vi "Main Page.vi"(8 "error in (no error)":errorcluster, 11 "Node Ptr":T1 format="%.0x") -> (0 "error out":errorcluster)   [LabVIEW 2019, in "SLSC EDS System Explorer.lvlib"]
uses:
  SLSC EDS System Explorer.lvlib
  <vilib>/NI VeriStand/Custom Device API/Custom Device Item Ref.ctl
  <vilib>/Utility/error.llb/DialogType.ctl
  <vilib>/Utility/miscctls.llb/LVStringsAndValuesArrayTypeDef_U16.ctl
  Shared/Constants.vi
  <vilib>/NI VeriStand/Custom Device API/Set Item Property (Variant).vi
  <vilib>/SLSC/Initialize Session with Devices.vi
  <vilib>/SLSC/Close Session.vi
  <vilib>/NI VeriStand/Custom Device API/Custom Device API.lvlib
  Shared/SLSC EDS Shared.lvlib
  SLSC UI API/SLSC Tree Control.lvlib
  SLSC CD API/SLSC CD System Explorer/SLSC CD System Explorer.lvlib
  Engine/SLSC EDS Engine.lvlib
  <vilib>/SLSC/SLSC.lvlib
  SLSC EDS API/SLSC EDS API.lvlib
  SLSC CD API/SLSC CD Engine/SLSC CD Engine.lvlib
panel:
  out "Custom Device State":string
  in  "Refresh page":bool
  out "SLSC Device Name":string
  out "State":u16(ring) items=["Not Configured", "Basic Configured"]
  out "Module Name":string
  in  "Help Button":bool
  out "Slot Number":i32
  out "CD Version":string caption="Version"
  in  "Header":cluster{"Section Name":string}={"Section Name"="SLSC EDS Custom Device"}
  in  "Name":string
  in  "SHDocVw.IWebBrowser":refnum<k7>(container)
  in  "Description":string
  in  "Modify Reset Value?":bool
  in  "I8":i8
  in  "U8":u8 format="%.0x"
  in  "I32":i32
  in  "U32":u32 format="%.0x"
  in  "U64":u64 format="%.0x"
  in  "I64":i64
  in  "DBL":dbl format="%#_16g"
  in  "Ring":u16(ring)
  in  "Add":bool
  in  "Remove":bool
  in  "Header 2":cluster{"Section Name":string}={"Section Name"="Custom Device Item Settings"}
  in  "Property tree":string[](tree)
  in  "Loop rate":u32
  in  "Apply Reset":bool
  in  "Apply Default":bool
  # "ms"
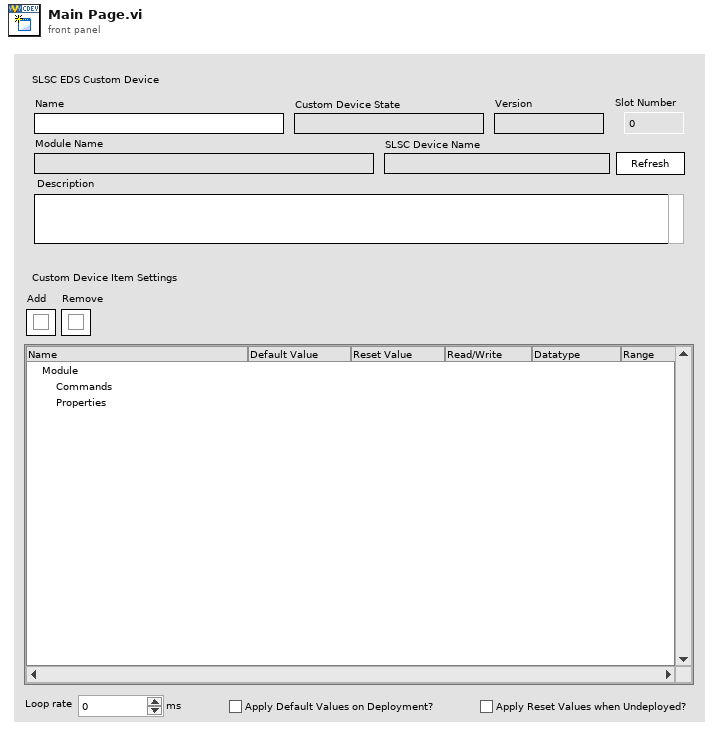
[diagram p1: front panel]
types:
  T1 = typedef "Custom Device API.lvlib/Custom Device Item Ref.ctl" = u64
  T2 = typedef "EDSjsonStructure.ctl" = cluster{"vendorNum":u32, "vendorName":string, "vendorPrefix":string, "productNum":u32, "productName":string, "capsVersion":string, "capsSpecVersion":u32, "capsSpecOldestCompatibleVersion":u32, "enums":T3[], "properties":T4[], "commands":T5[], "scales":T6[], "physicalChannels":T7[], "registerMap":cluster{"registers":T8[]}}
  T3 = typedef "enum.ctl" = cluster{"name":string, "description-en":string, "values":cluster{"name":string, "description-en":string, "value":i32}[]}
  T4 = typedef "property.ctl" = cluster{"name":string, "description-en":string, "documentation-en":string, "dataType":string, "bitfield":string, "access":string, "scale":string, "value":variant, "min":variant, "max":variant, "default value":variant}
  T5 = typedef "command.ctl" = cluster{"name":string, "description-en":string, "documentation-en":string, "startBitfield":string, "waitTimeInMs":i32, "doneBitfield":string, "doneInterrupt":string, "doneTimeoutInMs":i32, "value":variant}
  T6 = typedef "scale.ctl" = cluster{"name":string, "description-en":string, "m":dbl, "b":dbl, "forwardCoeffs":dbl[], "reverseCoeffs":dbl[], "coercion":string, "table":cluster{"scaled":dbl, "unscaled":dbl}[]}
  T7 = typedef "physicalChannel.ctl" = cluster{"name":string, "description-en":string, "commands":T5[], "properties":T4[]}
  T8 = typedef "register.ctl" = cluster{"name":string, "description-en":string, "access":string, "address":u32, "size":u32, "bitfields":cluster{"name":string, "description-en":string, "offset":u32, "size":u32, "signed":bool, "strobe":bool}[]}
  T9 = cluster{"Left Cell String":string, "Child Text":string[], "Child Tag":string, "Item Indent":i32, "Child Only?":bool, "Glyph Index":i32}[]
  T10 = typedef "LVStringsAndValuesArrayTypeDef_U16.ctl" = cluster{"String":string, "Value":u16}[]
  T11 = typedef "Custom Device API.lvlib/Custom Device Commands.ctl" = enum16{"Default", "Item renamed", "Shutdown", "Dynamic button pressed"}
  T12 = typedef "Custom Device API.lvlib/Custom Device Item Info.ctl" = cluster{"Name":string, "Is Channel":bool, "GUID":string, "Is Waveform":bool}
  T13 = typedef "DialogType.ctl" = u16
  T14 = typedef "SLSC EDS Shared.lvlib/SLSC Static Settings.ctl" = cluster{"Properties":cluster{"Boolean Properties":cluster{"property":refnum<k21>, "Value":bool, "SLSC Item":refnum<k21>, "reset value":bool}[], "Double Properties":cluster{"property":refnum<k21>, "Double Write":dbl, "SLSC Item":refnum<k21>, "Double Reset Value":dbl}[], "I32 Properties":cluster{"property":refnum<k21>, "Int32 Write":i32, "SLSC Item":refnum<k21>, "Int32 Reset Value":i32}[], "I64 Properties":cluster{"property":refnum<k21>, "Int64 Write":i64, "SLSC Item":refnum<k21>, "Int64 Reset Value":i64}[], "String Properties":cluster{"property":refnum<k21>, "String Write":string, "SLSC Item":refnum<k21>, "String Reset Value":string}[], "U32 Properties":cluster{"property":refnum<k21>, "UInt32 Write":u32, "SLSC Item":refnum<k21>, "UInt32 Reset Value":u32}[], "U64 Properties":cluster{"property":refnum<k21>, "UInt64 Write":u64, "SLSC Item":refnum<k21>, "UInt64 Reset Value":u64}[]}, "Commands":T15[], "Reset Commands":T15[], "Apply Values on Deployment":bool, "Apply Reset on Undeployment":bool, "Change Commands":T15[]}
  T15 = typedef "SLSC CD Shared.lvlib/SLSC Dynamic Channel.ctl" = cluster{"SLSC Item":string, "property":string, "Data Type":T16}
  T16 = typedef "SLSC CD Shared.lvlib/SLSC Datatype.ctl" = enum16{"Bool", "Double", "I32", "I64", "String", "U32", "U64"}
  T17 = typedef "SLSC CD Shared.lvlib/SLSC Identification.ctl" = cluster{"vendorName":string, "productNum":u32, "capsVersion":string, "capsSpecVersion":u32, "productName":string, "vendorNum":u32, "vendorPrefix":string, "capsSpecOldestCompatibleVersion":u32}
  T18 = cluster{"Left Cell String":string, "Child Text":string[], "Child Tag":string, "Item Indent":i32, "Child Only?":bool, "Glyph Index":i32}
  T19 = cluster{"name":string, "description-en":string, "value":i32}[]
  T20 = typedef "LVPoint32TypeDef.ctl" = cluster{"Horizontal":i32, "Vertical":i32}
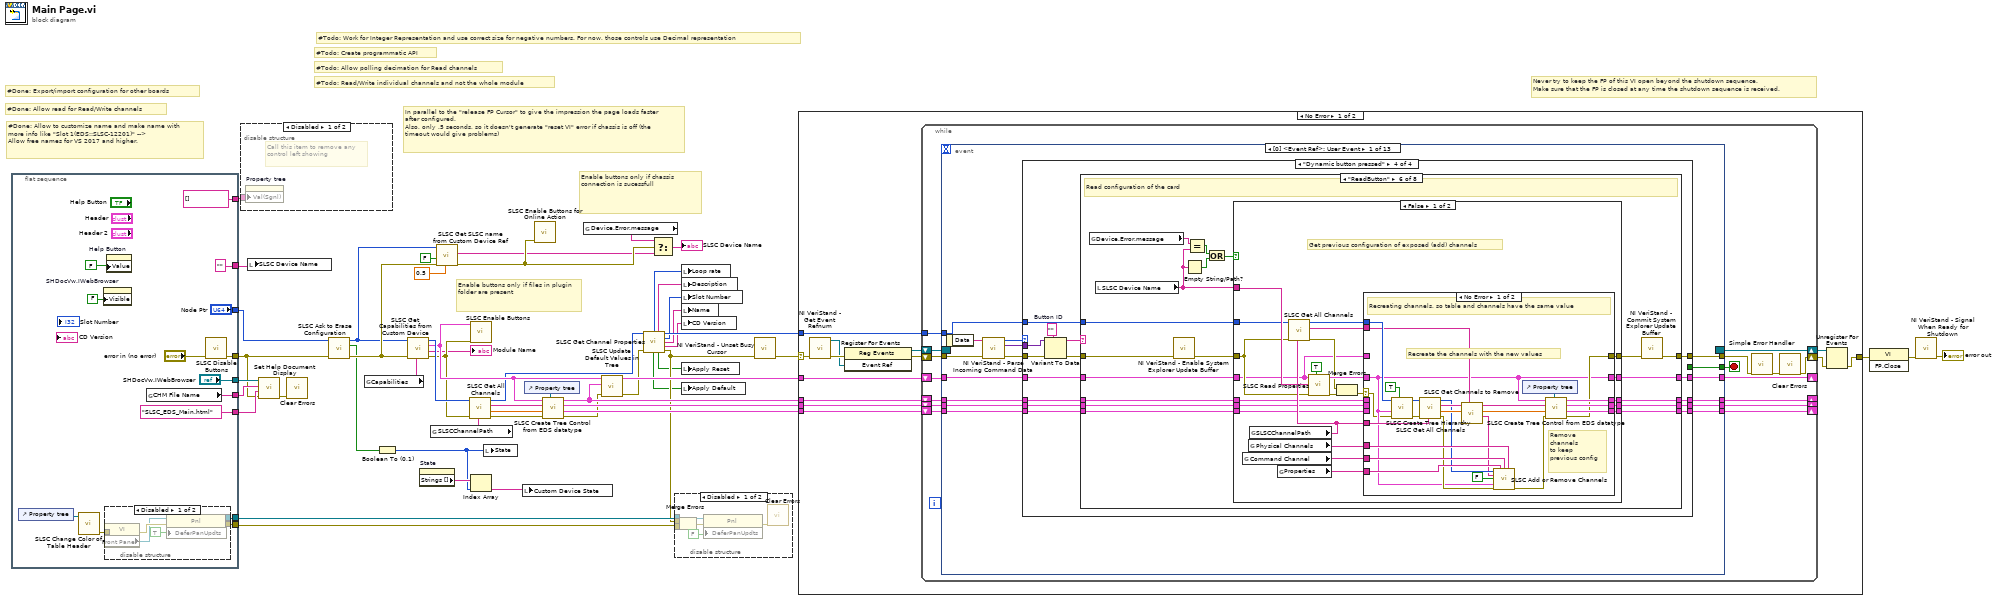
[diagram p0: block diagram]
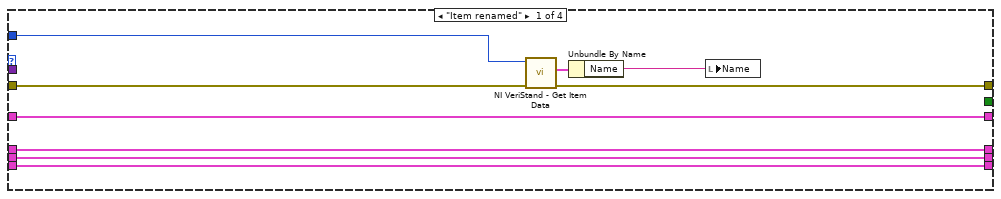
[diagram p5: hidden frame]
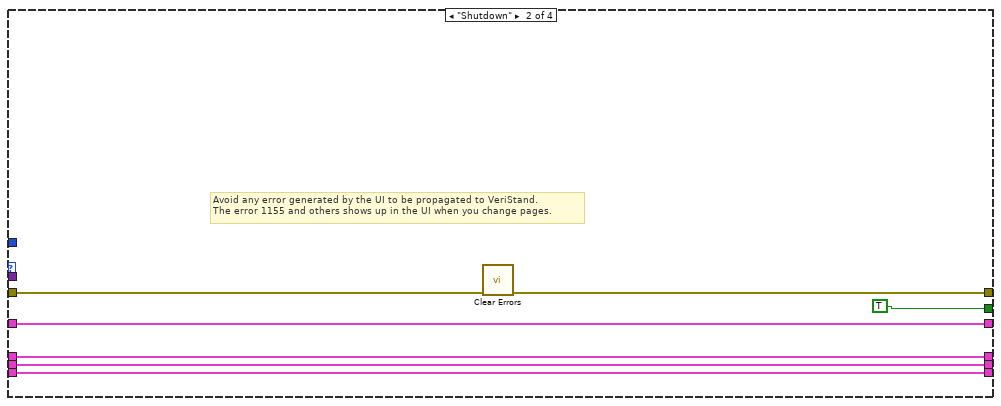
[diagram p6: hidden frame]
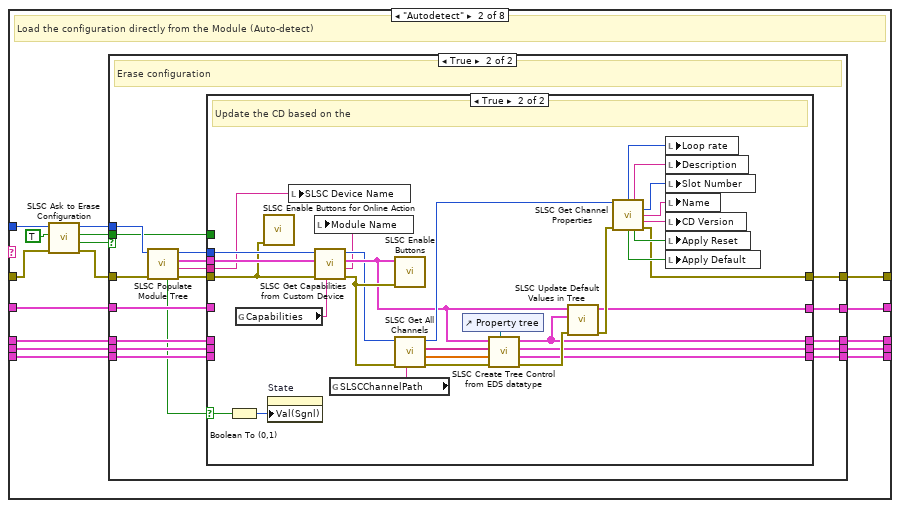
[diagram p9: hidden frame]
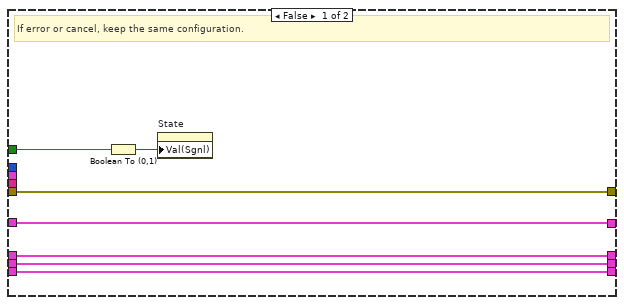
[diagram p11: hidden frame]
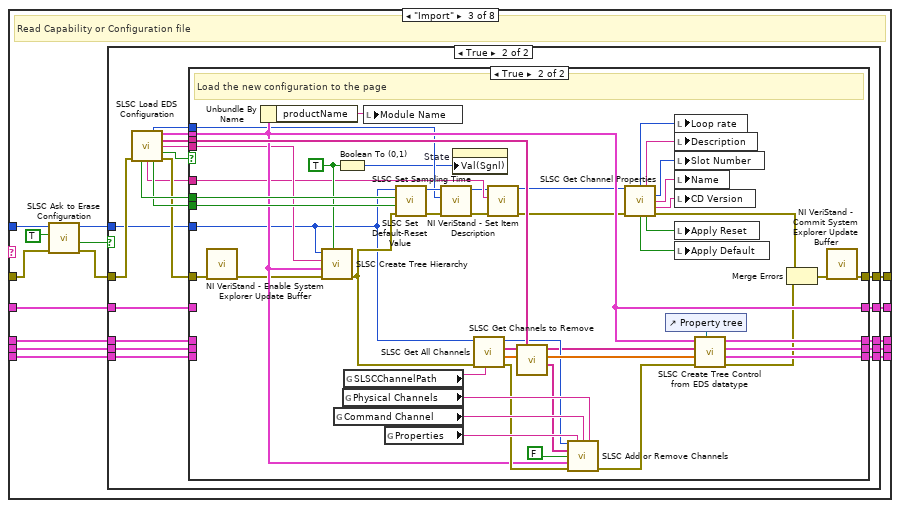
[diagram p12: hidden frame]
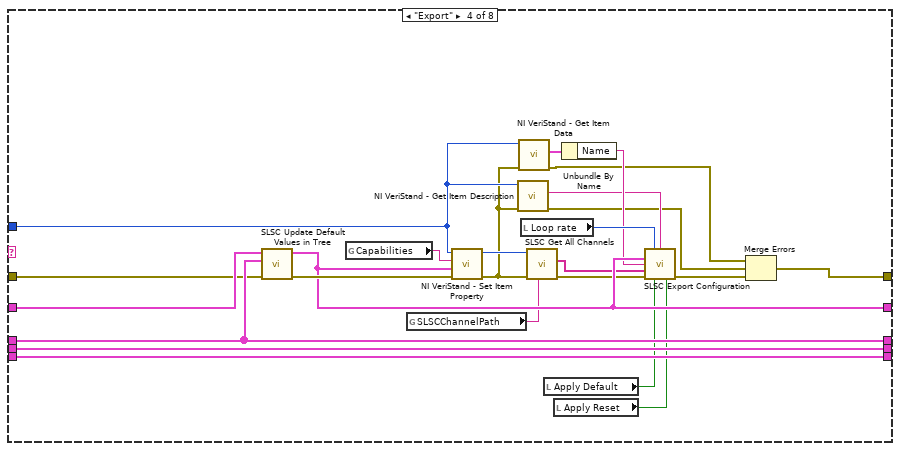
[diagram p15: hidden frame]
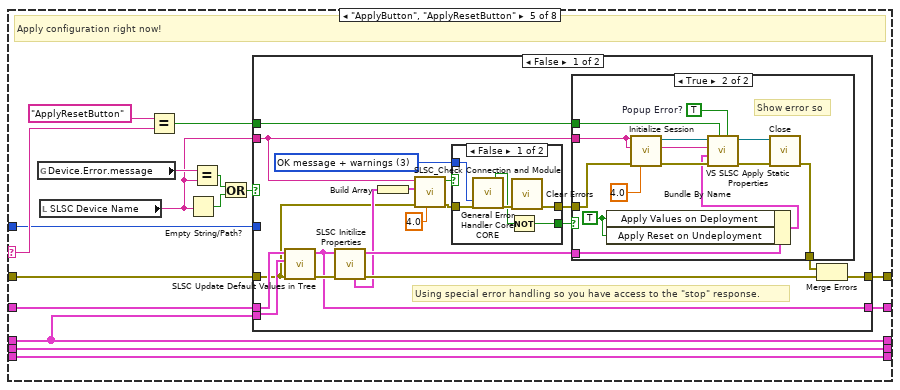
[diagram p16: hidden frame]
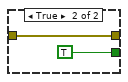
[diagram p18: hidden frame]
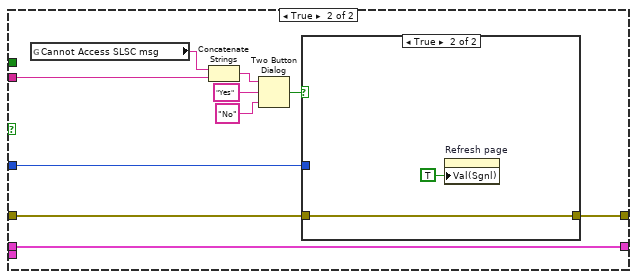
[diagram p19: hidden frame]
diagram:
  # "Enable buttons only if files in plugin folder are present"
  # "Enable buttons only if chassis connection is sucessfull"
  # "#Todo: Work for Integer Representation and use correct size for negative numbers. For now, those controls use Decimal representation"
  # "#Done: Allow to customize name and make name with more info like \"Slot 1(EDS::SLSC-12201)\" --> \nAllow free names for VS 2017 and higher."
  # "#Todo: Read/Write individual channels and not the whole module"
  # "In parallel to the \"release FP Cursor\" to give the impression the page loads faster after configured. \nAlso, only .5 seconds, so it doesn't generate \"reset VI\" error if chassis is off (the timeout would give problems)"
  # "Never try to keep the FP of this VI open beyond the shutdown sequence.\nMake sure that the FP is closed at any time the shutdown sequence is received."
  # "#Todo: Allow polling decimation for Read channels"
  # "#Done: Allow read for Read/Write channels"
  # "#Todo: Create programmatic API"
  # "#Done: Export/import configuration for other boards"
  n1 = flat-sequence {
    tunnel: ["Node Ptr"] -> w10
    tunnel: [w53] -> w11
    tunnel: ["SHDocVw.IWebBrowser"] -> w50
    tunnel: ["SLSC_EDS_Main.html" ("HTML File")] -> w49
    tunnel: [w63] -> w48
    tunnel: [string[] [] ("Property tree")] -> w43
    tunnel: ["" ("SLSC Module Name")] -> w42
    tunnel: [w57] -> w31
    tunnel: [w56] -> w30
    frame #0 {
      n2 = control-ref of="Property tree"() -> (w55:refnum<vi>)
      n3 = call "SLSC Change Color of Table Header.vi"("TreeControl in"=w55) -> ("error out"=w54:errorcluster)  [unwired: 10 in]
      n4 = property on="SHDocVw.IWebBrowser" class="AXCont"("Visible"=FALSE) -> ()  [unwired: 2 in, 2 out]
      n5 = disable-structure shown="Disabled" {
        disable-tunnel: [w70 _] -> w57
        disable-tunnel: [w69 _] -> w56
        disable-tunnel: w54 -> [w67 _]
        frame Disabled {
          n6 = property class="VI"(error in=w67) -> (error out=w72:errorcluster, "Front Panel"=w68:refnum<vi>)  [unwired: 1 in, 1 out]
          n7 = property class="Pnl"(reference=w68, error in=w72, "DeferPanUpdts"=TRUE ("Defer Panel Updates")) -> (reference out=w70:refnum<vi>, error out=w69:errorcluster)
        }
        frame Enabled {
        }
      }
      n8 = property on="Help Button" class="Bool (strict)"("Value"=FALSE ("Visible")) -> ()  [unwired: 2 in, 2 out]
      n9 = global read "Constants.vi" "CHM File Name"() -> (w63:string)
      n10 = call "SLSC Disable Buttons.vi"("error in (no error)"="error in (no error)") -> ("error out"=w53:errorcluster)  [unwired: 10 in]
    }
  }
  n11 = disable-structure shown="Disabled" {
    disable-tunnel: w43 -> [w73 _]
    frame Disabled {
      # "Call this item to remove any control left showing"
      n12 = property on="Property tree" class="Tree (strict)"("Val(Sgnl)"=w73) -> ()  [unwired: 2 in, 2 out]
    }
    frame Enabled {
    }
  }
  n13 = local write "SLSC Device Name"(w42) -> ()
  n14 = call "Set Help Document Display.vi"("error in (no error)"=w11, "HTML File"=w49, "Main CHM File"=w48, "SHDocVw.IWebBrowser2"=w50) -> ("error out"=w29:errorcluster)  [unwired: 7 in]
  n15 = call <vilib>:"Clear Errors.vi"("error in (no error)"=w29) -> ()  [unwired: 1 in, 6 out]
  n16 = call "SLSC Ask to Erase Configuration.vi"("error in (no error)"=w11, "Device Item Ref in"=w10) -> ("error out"=w41:errorcluster, "initialized?"=w9:bool, "Item Ref out"=w40:T1)  [unwired: 6 in, 1 out]
  n17 = global read "Constants.vi" "Capabilities"() -> (w32:string)
  n18 = Boolean To (0,1)(Boolean=w9) -> (0, 1=w2:i16)
  n19 = call "SLSC Get Capabilities from Custom Device.vi"("Property Name"=w32, "error in (no error)"=w41, "Device Item Ref in"=w40) -> ("error out"=w28:errorcluster, "Product Name"=→"Module Name":string, "data"=w34:T2, "Item Ref out"=w38:T1)  [unwired: 3 in, 2 out]
  n20 = property on="State" class="Ring (strict)"() -> ("Strings []"=w3:string[])  [unwired: 2 in, 2 out]
  n21 = global read "Constants.vi" "SLSCChannelPath"() -> (w33:string)
  n22 = call "SLSC Get SLSC name from Custom Device Ref.vi"("connect timeout"=0.5, "error in (no error)"=w41, "Wait for mDSN?"=FALSE, "Item Ref in"=w40) -> ("error out"=w15:errorcluster, "SLSC Module Name"=w14:string)  [unwired: 4 in, 2 out]
  n23 = call "SLSC Get All Channels.vi"("SLSCChannelPath"=w33, "error in (no error)"=w28, "Item Ref in"=w38) -> ("error out"=w37:errorcluster, "Channel Values"=w35:dbl[], "TreeItem Channels"=w36:string[], "Item Ref out"=w16:T1)  [unwired: 5 in]
  n24 = call "SLSC Enable Buttons.vi"("error in (no error)"=w28, "data"=w34) -> ()  [unwired: 10 in]
  n25 = Index Array(array=w3, index=w2) -> (element=w1:string)
  n26 = local write "State"(w2) -> ()
  n27 = local write "Custom Device State"(w1) -> ()
  n28 = control-ref of="Property tree"() -> (w39:refnum<vi>)
  n29 = call "SLSC Enable Buttons for Online Action.vi"("error in (no error)"=w15) -> ()  [unwired: 11 in]
  n30 = call "SLSC Create Tree Control from EDS datatype.vi"("Property Tree"=w39, "error in (no error)"=w37, "Channel Values"=w35, "Properties to enable"=w36, "SLSC EDS module"=w34) -> ("error out"=w24:errorcluster, "Enum Strings"=w44:cluster{"name":string, string}[], "Enums"=w45:T3[], "SLSC Output Tree"=w46:T9)  [unwired: 3 in]
  n31 = global read "Constants.vi" "Device.Error.message"() -> (w12:string)
  n32 = call "SLSC Update Default Values in Tree.vi"("error in (no error)"=w24, "SLSC Output Tree"=w46, "SLSC EDS module in"=w34) -> ("error out"=w23:errorcluster, "SLSC EDS module out"=w47:T2)  [unwired: 7 in]
  n33 = call "SLSC Get Channel Properties.vi"("Node Ptr"=w16, "error in (no error)"=w23) -> ("Loop time (ms)"=w17:u32, "Description"=w19:string, "Section Ref out"=w22:T1, "Module Number"=w6:i32, "Name"=w18:string, "Device Version"=w5:string, "Default Value"=w21:bool, "Reset Value"=w20:bool, "error out"=w25:errorcluster)  [unwired: 5 in]
  n34 = Select(t=w12, s=w15, f=w14) -> (s? t:f=→"SLSC Device Name":string)
  n35 = disable-structure shown="Disabled" {
    disable-tunnel: w31 -> [w77 _]
    disable-tunnel: w30 -> [w76 _]
    disable-tunnel: w25 -> [w75 _]
    frame Disabled {
      n36 = Merge Errors(w75, w76) -> (w78:errorcluster)
      n37 = property class="Pnl"(reference=w77, error in=w78, "DeferPanUpdts"=FALSE ("Defer Panel Updates")) -> (error out=w74:errorcluster)  [unwired: 1 out]
      n38 = call <vilib>:"Clear Errors.vi"("error in (no error)"=w74) -> ()  [unwired: 1 in, 6 out]
    }
    frame Enabled {
    }
  }
  n39 = local write "Loop rate"(w17) -> ()
  n40 = local write "Description"(w19) -> ()
  n41 = local write "Slot Number"(w6) -> ()
  n42 = local write "Name"(w18) -> ()
  n43 = local write "CD Version"(w5) -> ()
  n44 = local write "Apply Reset"(w20) -> ()
  n45 = local write "Apply Default"(w21) -> ()
  n46 = call <vilib>:"NI VeriStand - Unset Busy Cursor.vi"("error in (no error)"=w25) -> ("error out"=w27:errorcluster)  [unwired: 10 out]
  n47 = case shown="No Error" w27 {
    selector: w27 -> [w84 w989]
    tunnel: [w89 w990] -> w52
    tunnel: w22 -> [w85 _]
    tunnel: w47 -> [w83 _]
    tunnel: w46 -> [w82 _]
    tunnel: w45 -> [w81 _]
    tunnel: w44 -> [w80 _]
    frame No Error {
      n48 = call <vilib>:"NI VeriStand - Get Event Refnum.vi"("error in (no error)"=w84) -> ("error out"=w92:errorcluster, "Event Ref"=w88:refnum<user-event>)  [unwired: 9 out]
      n49 = register-events(error in=w92, w88) -> (reference out=w86:refnum<event-registration>, error out=w87:errorcluster)  [unwired: 1 in]
      n50 = while {
        tunnel: w85 -> [w104]
        shift-right: [w102] -> w90
        shift-left: w87 -> [w107]
        shift-right: [w108] -> w91
        shift-left: w86 -> [w106]
        shift-right: [w98] -> _
        shift-left: w82 -> [w100]
        shift-right: [w96] -> _
        shift-left: w83 -> [w101]
        shift-right: [w95] -> _
        shift-left: w81 -> [w99]
        shift-right: [w94] -> _
        shift-left: w80 -> [w97]
        stop <- w105 stop-if-true
        n51 = event shown="[0] <Event Ref>: User Event" {
          selector: w106 -> [_ _ _ w855 _ _ _ _ _ _ _ _ _]
          dyn-events: [_ _ _ w855 _ _ _ _ _ _ _ _ _] -> w108
          timeout: _ -> [_ _ _ _ _ _ _ _ _ _ _ _ _]
          tunnel: w107 -> [w124 w549 w828 w848 w856 w897 w913 w919 w926 w936 w943 w945 w986]
          tunnel: [w120 _ _ _ _ _ _ _ _ _ _ _ _] -> w105
          tunnel: [w119 w549 w827 w847 w861 w896 w913 w919 w920 w935 w942 w946 w972] -> w93
          tunnel: w104 -> [w118 _ _ _ w857 w890 _ _ w927 w934 w944 w955 w969]
          tunnel: w101 -> [w116 w548 w835 w854 w860 _ w912 w916 w924 w932 w939 w958 w978]
          tunnel: w100 -> [w115 w551 w836 w853 w863 _ w911 w917 w928 w933 w940 w963 w984]
          tunnel: w99 -> [w112 w544 w837 w850 w858 _ w909 w914 w922 w930 w937 w956 w975]
          tunnel: [w113 w551 w836 w853 w863 w873 w911 w917 w928 w933 w940 w963 w971] -> w98
          tunnel: w97 -> [w111 w545 w838 w851 w859 _ w910 w915 w923 w931 w938 w957 w976]
          tunnel: [w114 w548 w835 w854 w860 w884 w912 w916 w924 w932 w939 w958 w970] -> w96
          tunnel: [w110 w544 w837 w850 w858 w872 w909 w914 w922 w930 w937 w956 w975] -> w95
          tunnel: [w109 w545 w838 w851 w859 w871 w910 w915 w923 w931 w938 w957 w976] -> w94
          event User Event {
            n52 = event-data() -> ("Data"=w123:string)  [unwired: 1 out]
            n53 = call <vilib>:"NI VeriStand - Parse Incoming Command Data.vi"("error in (no error)"=w124, "Incoming data"=w123) -> ("error out"=w122:errorcluster, "Outgoing data"=w117:variant, "Action"=w121:T11)  [unwired: 7 out]
            n54 = case shown="\"Dynamic button pressed\"" w121 {
              tunnel: w122 -> [w133 w134 w145 w160]
              tunnel: [_ TRUE _ _] -> w120
              tunnel: [w130 w136 w145 w155] -> w119
              tunnel: w118 -> [w132 _ _ w152]
              tunnel: w117 -> [_ _ _ w159]
              tunnel: w116 -> [w128 w135 w144 w153]
              tunnel: w115 -> [w127 w139 w143 w154]
              tunnel: [w128 w135 w144 w151] -> w114
              tunnel: [w127 w139 w143 w150] -> w113
              tunnel: w112 -> [w125 w137 w141 w149]
              tunnel: w111 -> [w126 w138 w142 w148]
              tunnel: [w125 w137 w141 w147] -> w110
              tunnel: [w126 w138 w142 w146] -> w109
              frame "Item renamed" {
                n55 = call <vilib>:"NI VeriStand - Get Item Data.vi"("error in (no error)"=w133, "Item Ref in"=w132) -> ("error out"=w130:errorcluster, "Item Info"=w131:T12)  [unwired: 8 out]
                n56 = Unbundle By Name(w131) -> ("Name"=w129:string)
                n57 = local write "Name"(w129) -> ()
              }
              frame "Shutdown" {
                # "Avoid any error generated by the UI to be propagated to VeriStand.\nThe error 1155 and others shows up in the UI when you change pages."
                n58 = call <vilib>:"Clear Errors.vi"("error in (no error)"=w134) -> ("error out"=w136:errorcluster)  [unwired: 1 in, 5 out]
              }
              frame "Default", Default {
              }
              frame "Dynamic button pressed" {
                w158 = ""  # Button ID
                n59 = Variant To Data(error in=w160, type=w158, Variant=w159) -> (data=w157:string, error out=w156:errorcluster)
                n60 = case shown="\"ReadButton\"" w157 {
                  selector: w157 -> [_ _ _ _ w373 _ w520 _]
                  tunnel: w156 -> [w165 w172 w246 w354 w370 w436 w521 w537]
                  tunnel: [w165 w173 w248 w337 w369 w434 w524 w536] -> w155
                  tunnel: w154 -> [w163 w177 w252 w356 w366 w446 w518 w534]
                  tunnel: w153 -> [w164 w174 w250 w355 w374 w445 w519 w535]
                  tunnel: w152 -> [_ w171 w245 w341 w368 w444 _ _]
                  tunnel: [w164 w178 w249 w350 w367 w442 w519 w535] -> w151
                  tunnel: [w163 w179 w256 w356 w366 w441 w518 w534] -> w150
                  tunnel: w149 -> [w162 w176 w253 w351 w365 w440 w516 w532]
                  tunnel: w148 -> [w161 w175 w251 w352 w364 w439 w517 w533]
                  tunnel: [w162 w180 w255 w351 w365 w438 w516 w532] -> w147
                  tunnel: [w161 w181 w254 w352 w364 w437 w517 w533] -> w146
                  frame Default {
                  }
                  frame "Autodetect" {
                    # "Load the configuration directly from the Module (Auto-detect)"
                    n61 = call "SLSC Ask to Erase Configuration.vi"("error in (no error)"=w172, "Ask to erase?"=TRUE, "Device Item Ref in"=w171) -> ("error out"=w168:errorcluster, "Erase Data?"=w167:bool, "initialized?"=w166:bool, "Item Ref out"=w170:T1)  [unwired: 5 in]
                    n62 = case shown="True" w167 {
                      tunnel: [w184 w200] -> w181
                      tunnel: [w185 w199] -> w180
                      tunnel: [w186 w198] -> w179
                      tunnel: [w183 w197] -> w178
                      tunnel: w177 -> [w186 w195]
                      tunnel: w176 -> [w185 w194]
                      tunnel: w175 -> [w184 w193]
                      tunnel: w174 -> [w183 w192]
                      tunnel: [w182 w190] -> w173
                      tunnel: w170 -> [_ w189]
                      tunnel: w168 -> [w182 w188]
                      tunnel: w166 -> [_ w187]
                      frame False {
                        # "You decided not to erase previous configuration"
                      }
                      frame True {
                        # "Erase configuration"
                        n63 = call "SLSC Populate Module Tree.vi"("error in (no error)"=w188, "Device Item Ref in"=w189) -> ("error out"=w201:errorcluster, "SLSC Module Name"=w196:string, "SLSC EDS module"=w203:T2, "Device Item Ref out"=w202:T1, "Initialized?"=w191:bool)  [unwired: 5 in]
                        n64 = case shown="True" w191 {
                          selector: w191 -> [_ w212]
                          tunnel: w203 -> [_ w226]
                          tunnel: w202 -> [_ w223]
                          tunnel: w201 -> [w206 w222]
                          tunnel: [w208 w221] -> w200
                          tunnel: [w209 w220] -> w199
                          tunnel: [w210 w219] -> w198
                          tunnel: [w207 w218] -> w197
                          tunnel: w196 -> [_ w215]
                          tunnel: [w206 w213] -> w190
                          tunnel: w195 -> [w210 _]
                          tunnel: w194 -> [w209 _]
                          tunnel: w193 -> [w208 _]
                          tunnel: w192 -> [w207 _]
                          tunnel: w187 -> [w205 _]
                          frame False {
                            # "If error or cancel, keep the same configuration."
                            n65 = Boolean To (0,1)(Boolean=w205) -> (0, 1=w204:i16)
                            n66 = property on="State" class="Ring (strict)"("Val(Sgnl)"=w204) -> ()  [unwired: 2 in, 2 out]
                          }
                          frame True {
                            # "Update the CD based on the"
                            n67 = Boolean To (0,1)(Boolean=w212) -> (0, 1=w211:i16)
                            n68 = global read "Constants.vi" "Capabilities"() -> (w232:string)
                            n69 = call "SLSC Enable Buttons for Online Action.vi"("error in (no error)"=w222) -> ()  [unwired: 11 in]
                            n70 = property on="State" class="Ring (strict)"("Val(Sgnl)"=w211) -> ()  [unwired: 2 in, 2 out]
                            n71 = local write "SLSC Device Name"(w215) -> ()
                            n72 = call "SLSC Get Capabilities from Custom Device.vi"("Property Name"=w232, "error in (no error)"=w222, "Default Value"=w226, "Device Item Ref in"=w223) -> ("error out"=w233:errorcluster, "Product Name"=w217:string, "data"=w230:T2, "Item Ref out"=w225:T1)  [unwired: 2 in, 2 out]
                            n73 = local write "Module Name"(w217) -> ()
                            n74 = global read "Constants.vi" "SLSCChannelPath"() -> (w231:string)
                            n75 = call "SLSC Enable Buttons.vi"("error in (no error)"=w233, "data"=w230) -> ()  [unwired: 10 in]
                            n76 = call "SLSC Get All Channels.vi"("SLSCChannelPath"=w231, "error in (no error)"=w233, "Item Ref in"=w225) -> ("error out"=w227:errorcluster, "Channel Values"=w229:dbl[], "TreeItem Channels"=w228:string[], "Item Ref out"=w234:T1)  [unwired: 5 in]
                            n77 = control-ref of="Property tree"() -> (w224:refnum<vi>)
                            n78 = call "SLSC Create Tree Control from EDS datatype.vi"("Property Tree"=w224, "error in (no error)"=w227, "Channel Values"=w229, "Properties to enable"=w228, "SLSC EDS module"=w230) -> ("error out"=w235:errorcluster, "Enum Strings"=w221:cluster{"name":string, string}[], "Enums"=w220:T3[], "SLSC Output Tree"=w219:T9)  [unwired: 3 in]
                            n79 = call "SLSC Update Default Values in Tree.vi"("error in (no error)"=w235, "SLSC Output Tree"=w219, "SLSC EDS module in"=w230) -> ("error out"=w236:errorcluster, "SLSC EDS module out"=w218:T2)  [unwired: 7 in]
                            n80 = call "SLSC Get Channel Properties.vi"("Node Ptr"=w234, "error in (no error)"=w236) -> ("Loop time (ms)"=w241:u32, "Description"=w239:string, "Module Number"=w216:i32, "Name"=w240:string, "Device Version"=w214:string, "Default Value"=w237:bool, "Reset Value"=w238:bool, "error out"=w213:errorcluster)  [unwired: 5 in, 1 out]
                            n81 = local write "Loop rate"(w241) -> ()
                            n82 = local write "Description"(w239) -> ()
                            n83 = local write "Slot Number"(w216) -> ()
                            n84 = local write "Name"(w240) -> ()
                            n85 = local write "CD Version"(w214) -> ()
                            n86 = local write "Apply Reset"(w238) -> ()
                            n87 = local write "Apply Default"(w237) -> ()
                          }
                        }
                      }
                    }
                  }
                  frame "Import" {
                    # "Read Capability or Configuration file"
                    n88 = call "SLSC Ask to Erase Configuration.vi"("error in (no error)"=w246, "Ask to erase?"=TRUE, "Device Item Ref in"=w245) -> ("error out"=w243:errorcluster, "Erase Data?"=w242:bool, "Item Ref out"=w244:T1)  [unwired: 5 in, 1 out]
                    n89 = case shown="True" w242 {
                      tunnel: [w259 w280] -> w256
                      tunnel: [w258 w279] -> w255
                      tunnel: [w257 w278] -> w254
                      tunnel: w253 -> [w258 w277]
                      tunnel: w252 -> [w259 w270]
                      tunnel: w251 -> [w257 w269]
                      tunnel: w250 -> [w261 w268]
                      tunnel: [w261 w267] -> w249
                      tunnel: [w260 w266] -> w248
                      tunnel: w243 -> [w260 w265]
                      tunnel: w244 -> [_ w264]
                      frame False {
                        # "Decided to not overwrite previous configuration"
                      }
                      frame True {
                        n90 = call "SLSC Load EDS Configuration.vi"("error in (no error)"=w265) -> ("Loop rate"=w275:u32, "SLSC EDS module out"=w281:T2, "Enable Channels"=w276:string[], "Custom Device Name"=w263:string, "Has capability?"=w271:bool, "Apply Default"=w274:bool, "Custom Device Description"=w262:string, "Apply Reset"=w273:bool, "error out"=w272:errorcluster)  [unwired: 5 in, 1 out]
                        n91 = case shown="True" w271 {
                          tunnel: w264 -> [_ w288]
                          tunnel: w281 -> [_ w306]
                          tunnel: [w286 w334] -> w280
                          tunnel: [w285 w333] -> w279
                          tunnel: [w284 w332] -> w278
                          tunnel: w277 -> [w285 _]
                          tunnel: [w283 w300] -> w266
                          tunnel: w276 -> [_ w322]
                          tunnel: w275 -> [_ w296]
                          tunnel: w274 -> [_ w317]
                          tunnel: w273 -> [_ w316]
                          tunnel: w272 -> [w283 w302]
                          tunnel: w270 -> [w286 _]
                          tunnel: w269 -> [w284 _]
                          tunnel: w268 -> [w282 _]
                          tunnel: [w282 w306] -> w267
                          tunnel: w263 -> [_ w294]
                          tunnel: w262 -> [_ w292]
                          frame False {
                            # "Error in reading the file. Don't change existent configuration."
                          }
                          frame True {
                            w303 = TRUE ("Initialized?")
                            # "Load the new configuration to the page"
                            n92 = call <vilib>:"NI VeriStand - Enable System Explorer Update Buffer.vi"("error in (no error)"=w302) -> ("error out"=w295:errorcluster)  [unwired: 10 in]
                            n93 = Unbundle By Name(w306) -> ("productName"=w318:string)
                            n94 = call "SLSC Create Tree Hierarchy.vi"("Initialized?"=w303, "error in (no error)"=w295, "SLSC EDS module"=w306, "Custom Device Name"=w294, "Item Ref in"=w288) -> ("error out"=w299:errorcluster)  [unwired: 5 in, 1 out]
                            n95 = global read "Constants.vi" "Command Channel"() -> (w327:string)
                            n96 = Boolean To (0,1)(Boolean=w303) -> (0, 1=w287:i16)
                            n97 = global read "Constants.vi" "Physical Channels"() -> (w329:string)
                            n98 = global read "Constants.vi" "SLSCChannelPath"() -> (w331:string)
                            n99 = local write "Module Name"(w318) -> ()
                            n100 = global read "Constants.vi" "Properties"() -> (w328:string)
                            n101 = call "SLSC Set Default-Reset Value.vi"("error in (no error)"=w299, "Apply Reset"=w316, "Apply Default"=w317, "Section Ref in"=w288) -> ("error out"=w298:errorcluster, "Item Ref out"=w297:T1)  [unwired: 6 in]
                            n102 = call "SLSC Set Sampling Time.vi"("error in (no error)"=w298, "Loop rate"=w296, "Section Ref in"=w297) -> ("error out"=w293:errorcluster, "Channel Ref out"=w291:T1)  [unwired: 7 in]
                            n103 = property on="State" class="Ring (strict)"("Val(Sgnl)"=w287) -> ()  [unwired: 2 in, 2 out]
                            n104 = call "SLSC Get All Channels.vi"("SLSCChannelPath"=w331, "error in (no error)"=w299, "Item Ref in"=w288) -> ("error out"=w307:errorcluster, "Channel Values"=w324:dbl[], "TreeItem Channels"=w325:string[], "Item Ref out"=w321:T1)  [unwired: 5 in]
                            n105 = call <vilib>:"NI VeriStand - Set Item Description.vi"("error in (no error)"=w293, "Description"=w292, "Item Ref in"=w291) -> ("error out"=w290:errorcluster, "Item Ref out"=w289:T1)  [unwired: 7 out]
                            n106 = call "SLSC Get Channels to Remove.vi"("Channels Created"=w322, "All Channel Values"=w324, "All Channels"=w325) -> ("Channels to be Deleted"=w320:string[], "Channel Values"=w323:dbl[], "Channels to be Added"=w319:string[])  [unwired: 6 in]
                            n107 = call "SLSC Add or Remove Channels.vi"("Section Ref in"=w321, "Properties"=w328, "Command Channel"=w327, "Physical Channels"=w329, "Property tree"=w320, "Add or Remove"=FALSE, "SLSC EDS module in"=w306, "error in (no error)"=w307) -> ("error out"=w305:errorcluster)  [unwired: 6 in, 1 out]
                            n108 = call "SLSC Get Channel Properties.vi"("Node Ptr"=w289, "error in (no error)"=w290) -> ("Loop time (ms)"=w308:u32, "Description"=w314:string, "Module Number"=w312:i32, "Name"=w315:string, "Device Version"=w311:string, "Default Value"=w310:bool, "Reset Value"=w313:bool, "error out"=w309:errorcluster)  [unwired: 5 in, 1 out]
                            n109 = control-ref of="Property tree"() -> (w330:refnum<vi>)
                            n110 = local write "Loop rate"(w308) -> ()
                            n111 = local write "Description"(w314) -> ()
                            n112 = local write "Slot Number"(w312) -> ()
                            n113 = local write "Name"(w315) -> ()
                            n114 = local write "CD Version"(w311) -> ()
                            n115 = local write "Apply Reset"(w313) -> ()
                            n116 = local write "Apply Default"(w310) -> ()
                            n117 = call "SLSC Create Tree Control from EDS datatype.vi"("Property Tree"=w330, "error in (no error)"=w305, "Channel Values"=w323, "Properties to enable"=w319, "SLSC EDS module"=w306) -> ("error out"=w304:errorcluster, "Enum Strings"=w332:cluster{"name":string, string}[], "Enums"=w333:T3[], "SLSC Output Tree"=w334:T9)  [unwired: 3 in]
                            n118 = Merge Errors(w309, w304) -> (w301:errorcluster)
                            n119 = call <vilib>:"NI VeriStand - Commit System Explorer Update Buffer.vi"("error in (no error)"=w301) -> ("error out"=w300:errorcluster)  [unwired: 10 in]
                          }
                        }
                      }
                    }
                  }
                  frame "Export" {
                    n120 = call "SLSC Update Default Values in Tree.vi"("error in (no error)"=w354, "SLSC Output Tree"=w356, "SLSC EDS module in"=w355) -> ("error out"=w357:errorcluster, "SLSC EDS module out"=w350:T2)  [unwired: 7 in]
                    n121 = global read "Constants.vi" "Capabilities"() -> (w358:string)
                    n122 = global read "Constants.vi" "SLSCChannelPath"() -> (w349:string)
                    n123 = call-poly <vilib>:"NI VeriStand - Set Item Property.vi"("error in (no error)"=w357, "Value"=w350, "Property Name"=w358, "Item Ref in"=w341) -> ("error out"=w340:errorcluster, "Item Ref out"=w348:T1)  [unwired: 5 in, 1 out]
                    n124 = call <vilib>:"NI VeriStand - Get Item Description.vi"("error in (no error)"=w340, "Item Ref in"=w341) -> ("error out"=w335:errorcluster, "Description"=w338:string)  [unwired: 6 in, 2 out]
                    n125 = call <vilib>:"NI VeriStand - Get Item Data.vi"("error in (no error)"=w340, "Item Ref in"=w341) -> ("error out"=w336:errorcluster, "Item Info"=w342:T12)  [unwired: 8 out]
                    n126 = local read "Loop rate"() -> (w345:u32)
                    n127 = call "SLSC Get All Channels.vi"("SLSCChannelPath"=w349, "error in (no error)"=w340, "Item Ref in"=w348) -> ("error out"=w346:errorcluster, "TreeItem Channels"=w347:string[])  [unwired: 5 in, 2 out]
                    n128 = local read "Apply Default"() -> (w344:bool)
                    n129 = local read "Apply Reset"() -> (w343:bool)
                    n130 = Unbundle By Name(w342) -> ("Name"=w339:string)
                    n131 = call "SLSC Export Configuration.vi"("Loop rate"=w345, "Description"=w338, "SLSC EDS module in"=w350, "Custom Device Name"=w339, "Channels to Enable"=w347, "error in (no error)"=w346, "Apply Default"=w344, "Apply Reset"=w343) -> ("error out"=w353:errorcluster)  [unwired: 7 in]
                    n132 = Merge Errors(w336, w335, w353) -> (w337:errorcluster)
                  }
                  frame "ApplyButton", "ApplyResetButton" {
                    # "Apply configuration right now!"
                    n133 = global read "Constants.vi" "Device.Error.message"() -> (w362:string)
                    n134 = local read "SLSC Device Name"() -> (w360:string)
                    n135 = Equal?(x="ApplyResetButton", y=w373) -> (x = y?=w372:bool)
                    n136 = Empty String/Path?(string/path=w360) -> (empty?=w363:bool)
                    n137 = Equal?(x=w362, y=w360) -> (x = y?=w361:bool)
                    n138 = Or(x=w361, y=w363) -> (x .or. y?=w359:bool)
                    n139 = case shown="False" w359 {
                      tunnel: w366 -> [w393 _]
                      tunnel: w374 -> [w385 w419]
                      tunnel: w372 -> [w392 _]
                      tunnel: w370 -> [w380 w424]
                      tunnel: [w390 w420] -> w369
                      tunnel: w360 -> [w384 w425]
                      tunnel: w368 -> [_ w423]
                      tunnel: [w386 w419] -> w367
                      frame False {
                        w375 = T13 3 items=["no dialog", "OK message", "continue or stop message", "OK message + warnings", "continue/stop + warnings"] ("type of dialog (OK msg:1)")
                        # "Using special error handling so you have access to the \"stop\" response."
                        n140 = call "SLSC Update Default Values in Tree.vi"("error in (no error)"=w380, "SLSC Output Tree"=w393, "SLSC EDS module in"=w385) -> ("error out"=w391:errorcluster, "SLSC EDS module out"=w386:T2)  [unwired: 7 in]
                        n141 = call "SLSC Initilize Properties.vi"("error in (no error)"=w391, "Capabilities"=w386) -> ("error out"=w389:errorcluster, "Configuration Data"=w388:T14, "Identification"=w383:T17)  [unwired: 5 in, 2 out]
                        n142 = Build Array(w383) -> (w382:T17[])
                        n143 = call "SLSC_Check Connection and Module.vi"("Connect timeout (s)"=4.0 ("connect timeout (10 sec)"), "error in (no error)"=w380, "Supported Modules"=w382, "devices"=w384) -> ("error out"=w378:errorcluster, "Device Found?"=w379:bool)  [unwired: 6 in]
                        n144 = case shown="False" w379 {
                          tunnel: [w408 TRUE ("T button?")] -> w377
                          tunnel: w378 -> [w412 w414]
                          tunnel: [w413 w414] -> w376
                          tunnel: w375 -> [w410 _]
                          frame False {
                            n145 = call <vilib>:"General Error Handler Core CORE.vi"("type of dialog (OK msg:1)"=w410, "error in (no error)"=w412) -> ("stop event propagated"=w409:bool, "error out"=w411:errorcluster)  [unwired: 12 in, 4 out]
                            n146 = Not(x=w409) -> (.not. x?=w408:bool)
                            n147 = call <vilib>:"Clear Errors.vi"("error in (no error)"=w411) -> ("error out"=w413:errorcluster)  [unwired: 5 in, 1 out]
                          }
                          frame True {
                          }
                        }
                        n148 = case shown="True" w377 {
                          tunnel: w392 -> [_ w402]
                          tunnel: w388 -> [_ w400]
                          tunnel: [w394 w397] -> w387
                          tunnel: w384 -> [_ w396]
                          tunnel: w376 -> [w394 w395]
                          frame False {
                            # "Avoid messaging incorrect board.\nAnd we ask just in case the user is \nsure the board is correct, just happen\nto not match the Board number"
                          }
                          frame True {
                            w398 = TRUE ("Apply Values on Deployment")
                            w401 = TRUE  # Popup Error?
                            # "Show error so"
                            n149 = Bundle By Name(cluster=w400, "Apply Values on Deployment"=w398, "Apply Reset on Undeployment"=w398) -> (w399:T14)
                            n150 = call-poly <vilib>:"Initialize Session.vi"("devices"=w396, "error in (no error)"=w395, "connect timeout (60 sec)"=4.0 ("connect timeout (10 sec)")) -> ("session out"=w406:refnum<k21>, "error out"=w407:errorcluster)  [unwired: 11 in]
                            n151 = call "VS SLSC Apply Static Properties.vi"("Popup Error?"=w401, "Reset?"=w402, "error in (no error)"=w407, "Configuration Data"=w399, "SLSC Module Name in"=w396, "Refnum in"=w406) -> ("error out"=w404:errorcluster, "Refnum out"=w403:refnum<k21>)  [unwired: 3 in, 1 out]
                            n152 = call-poly <vilib>:"Close.vi"("session in"=w403, "error in (no error)"=w404) -> ("error out"=w397:errorcluster)  [unwired: 13 in]
                          }
                        }
                        n153 = Merge Errors(w387, w389) -> (w390:errorcluster)
                      }
                      frame True {
                        n154 = global read "Constants.vi" "Cannot Access SLSC msg"() -> (w417:string)
                        n155 = Concatenate Strings(w417, w425) -> (w422:string)
                        n156 = Two Button Dialog(message=w422, 1:"No" ("F button name (\"Cancel\")"), 2:"Yes" ("F button name (\"Cancel\")")) -> (T button?=w421:bool)
                        n157 = case shown="True" w421 {
                          tunnel: w424 -> [w426 w428]
                          tunnel: w423 -> [_ _]
                          tunnel: [w426 w428] -> w420
                          frame False {
                          }
                          frame True {
                            n158 = property on="Refresh page" class="Bool (strict)"("Val(Sgnl)"=TRUE ("Value (Signaling)")) -> ()  [unwired: 2 in, 2 out]
                          }
                        }
                      }
                    }
                  }
                  frame "ReadButton" {
                    # "Read configuration of the card"
                    n159 = global read "Constants.vi" "Device.Error.message"() -> (w431:string)
                    n160 = local read "SLSC Device Name"() -> (w430:string)
                    n161 = call <vilib>:"NI VeriStand - Enable System Explorer Update Buffer.vi"("error in (no error)"=w436) -> ("error out"=w435:errorcluster)  [unwired: 10 in]
                    n162 = Empty String/Path?(string/path=w430) -> (empty?=w443:bool)
                    n163 = Equal?(x=w431, y=w430) -> (x = y?=w429:bool)
                    n164 = Or(x=w429, y=w443) -> (x .or. y?=w432:bool)
                    n165 = case shown="False" w432 {
                      tunnel: w446 -> [w450 w505]
                      tunnel: w445 -> [w451 w506]
                      tunnel: w435 -> [w457 w511]
                      tunnel: [w454 w507] -> w433
                      tunnel: w430 -> [w469 w512]
                      tunnel: w444 -> [w464 w510]
                      tunnel: [w452 w506] -> w442
                      tunnel: [w468 w505] -> w441
                      tunnel: w440 -> [w449 w503]
                      tunnel: w439 -> [w448 w502]
                      tunnel: [w460 w503] -> w438
                      tunnel: [w459 w502] -> w437
                      frame False {
                        # "Get previous configuration of exposed (add) channels"
                        n166 = global read "Constants.vi" "Command Channel"() -> (w465:string)
                        n167 = global read "Constants.vi" "Physical Channels"() -> (w467:string)
                        n168 = global read "Constants.vi" "SLSCChannelPath"() -> (w463:string)
                        n169 = global read "Constants.vi" "Properties"() -> (w466:string)
                        n170 = call "SLSC Get All Channels.vi"("SLSCChannelPath"=w463, "error in (no error)"=w457, "Item Ref in"=w464) -> ("error out"=w455:errorcluster, "TreeItem Channels"=w461:string[], "Item Ref out"=w462:T1)  [unwired: 5 in, 1 out]
                        n171 = call "SLSC Read Properties.vi"("Default Only?"=TRUE ("Read Only?"), "error in (no error)"=w457, "SLSC Device"=w469, "SLSC EDS module in"=w451) -> ("error out"=w456:errorcluster, "SLSC EDS module out"=w458:T2)  [unwired: 6 in]
                        n172 = Merge Errors(w455, w456) -> (w453:errorcluster)
                        n173 = case shown="No Error" w453 {
                          selector: w453 -> [w470 w498]
                          tunnel: [w494 w497] -> w468
                          tunnel: w467 -> [w491 _]
                          tunnel: w466 -> [w490 _]
                          tunnel: w465 -> [w489 _]
                          tunnel: w463 -> [w483 _]
                          tunnel: w462 -> [w482 _]
                          tunnel: w461 -> [w481 _]
                          tunnel: [w476 w496] -> w460
                          tunnel: [w475 w495] -> w459
                          tunnel: w458 -> [w471 _]
                          tunnel: [w472 w498] -> w454
                          tunnel: [w471 w499] -> w452
                          tunnel: w451 -> [_ w499]
                          tunnel: w450 -> [_ w497]
                          tunnel: w449 -> [_ w496]
                          tunnel: w448 -> [_ w495]
                          frame No Error {
                            # "Remove \nchannels\nto keep \nprevious config"
                            # "Recreate the channels with the new values"
                            # "Recreating channels, so table and channels have the same value"
                            n174 = call "SLSC Create Tree Hierarchy.vi"("Initialized?"=TRUE, "error in (no error)"=w470, "SLSC EDS module"=w471, "Item Ref in"=w482) -> ("error out"=w487:errorcluster, "Parent Ref out"=w486:T1)  [unwired: 6 in]
                            n175 = call "SLSC Get All Channels.vi"("SLSCChannelPath"=w483, "error in (no error)"=w487, "Item Ref in"=w486) -> ("error out"=w474:errorcluster, "Channel Values"=w484:dbl[], "TreeItem Channels"=w485:string[], "Item Ref out"=w479:T1)  [unwired: 5 in]
                            n176 = call "SLSC Get Channels to Remove.vi"("Channels Created"=w481, "All Channel Values"=w484, "All Channels"=w485) -> ("Channels to be Deleted"=w478:string[], "Channel Values"=w480:dbl[], "Channels to be Added"=w477:string[])  [unwired: 6 in]
                            n177 = call "SLSC Add or Remove Channels.vi"("Section Ref in"=w479, "Properties"=w490, "Command Channel"=w489, "Physical Channels"=w491, "Property tree"=w478, "Add or Remove"=FALSE, "SLSC EDS module in"=w471, "error in (no error)"=w474) -> ("error out"=w473:errorcluster)  [unwired: 6 in, 1 out]
                            n178 = control-ref of="Property tree"() -> (w493:refnum<vi>)
                            n179 = call "SLSC Create Tree Control from EDS datatype.vi"("Property Tree"=w493, "error in (no error)"=w473, "Channel Values"=w480, "Properties to enable"=w477, "SLSC EDS module"=w471) -> ("error out"=w472:errorcluster, "Enum Strings"=w475:cluster{"name":string, string}[], "Enums"=w476:T3[], "SLSC Output Tree"=w494:T9)  [unwired: 3 in]
                          }
                          frame Error {
                            # "If error, don't change state and report the error (outside)"
                          }
                        }
                      }
                      frame True {
                        n180 = global read "Constants.vi" "Cannot Access SLSC msg"() -> (w501:string)
                        n181 = Concatenate Strings(w501, w512) -> (w509:string)
                        n182 = Two Button Dialog(message=w509, 1:"No" ("F button name (\"Cancel\")"), 2:"Yes" ("F button name (\"Cancel\")")) -> (T button?=w508:bool)
                        n183 = case shown="False" w508 {
                          tunnel: w511 -> [w513 w515]
                          tunnel: w510 -> [_ _]
                          tunnel: [w513 w515] -> w507
                          frame False {
                          }
                          frame True {
                            n184 = property on="Refresh page" class="Bool (strict)"("Val(Sgnl)"=TRUE ("Value (Signaling)")) -> ()  [unwired: 2 in, 2 out]
                          }
                        }
                      }
                    }
                    n185 = call <vilib>:"NI VeriStand - Commit System Explorer Update Buffer.vi"("error in (no error)"=w433) -> ("error out"=w434:errorcluster)  [unwired: 10 in]
                  }
                  frame "Diagram", "Pinout" {
                    # "Open and forget..."
                    n186 = vi-ref "SLSC Show Pinout.vi"() -> (w522:refnum<vi>)
                    n187 = property class="VI Interface Type 13"(reference=w522) -> ("Name"=w523:string)  [unwired: 1 in, 2 out]
                    n188 = Unbundle By Name(w519) -> ("vendorPrefix"=w529:string, "productNum"=w528:u32)
                    n189 = Open VI Reference(type specifier VI Refnum (for type only)=w522, vi path=w523, options=128, error in (no error)=w521) -> (vi reference=w530:refnum<vi>, error out=w526:errorcluster)  [unwired: 2 in]
                    n190 = call-by-ref "Start Asynchronous Call"(reference=w530, error in=w526, "Type"=w520, "number"=w528, "Vendor Name"=w529) -> (reference out=w527:refnum<vi>, error out=w525:errorcluster)  [unwired: 9 in]
                    n191 = Close Reference(reference=w527, error in (no error)=w525) -> (error out=w524:errorcluster)
                  }
                  frame "HelpButton" {
                    # "Show Help Page"
                    n192 = property on="SHDocVw.IWebBrowser" class="AXCont"(error in=w537) -> (error out=w538:errorcluster, "Visible"=w540:bool)  [unwired: 1 in, 1 out]
                    n193 = Not(x=w540) -> (.not. x?=w539:bool)
                    n194 = property on="SHDocVw.IWebBrowser" class="AXCont"(error in=w538, "Visible"=w539) -> (error out=w536:errorcluster)  [unwired: 1 in, 1 out]
                  }
                }
              }
            }
          }
          event "Property tree": Value Change {
            n195 = event-data() -> ()  [unwired: 2 out]
            n196 = control-ref of="Modify Reset Value?"() -> (w550:refnum<vi>)
            n197 = control-ref of="DBL"() -> (w559:refnum<vi>)
            n198 = control-ref of="I8"() -> (w557:refnum<vi>)
            n199 = control-ref of="I32"() -> (w552:refnum<vi>)
            n200 = control-ref of="I64"() -> (w553:refnum<vi>)
            n201 = control-ref of="U8"() -> (w554:refnum<vi>)
            n202 = control-ref of="U32"() -> (w555:refnum<vi>)
            n203 = control-ref of="U64"() -> (w556:refnum<vi>)
            n204 = control-ref of="Ring"() -> (w558:refnum<vi>)
            n205 = Array Size(array="Property tree") -> (size(s)=w547:i32)
            n206 = Equal To 0?(x=w547) -> (x = 0?=w542:bool)
            n207 = Not Equal?(x=w547, y=1 ("x")) -> (x != y?=w546:bool)
            n208 = case shown="False" w542 {
              tunnel: "Property tree" -> [w565 _]
              tunnel: w551 -> [w566 _]
              tunnel: w544 -> [w575 _]
              tunnel: w556 -> [w576 w817]
              tunnel: w555 -> [w582 w818]
              tunnel: w554 -> [w577 w819]
              tunnel: w553 -> [w578 w820]
              tunnel: w552 -> [w579 w821]
              tunnel: w557 -> [w580 w822]
              tunnel: w558 -> [w583 w823]
              tunnel: w559 -> [w581 w824]
              tunnel: w545 -> [w572 _]
              tunnel: "Modify Reset Value?" -> [w568 _]
              tunnel: w550 -> [w569 w815]
              tunnel: w546 -> [w567 _]
              frame False {
                # "Use the default control based on the first selection"
                # "Only allow to modify the value of 1 selection, otherwise hide control."
                n209 = Index Array(array=w565) -> (element=w574:string)  [unwired: 1 in]
                n210 = call "SLSC Search Item in Tree Control.vi"("SLSC Output Tree"=w566, "Item Tag"=w574) -> ("Item"=w573:T18)  [unwired: 10 in, 3 out]
                n211 = call "SLSC Get Items from Tree Control.vi"("Item"=w573) -> ("Value"=w564:string, "Datatype"=w561:string, "Type of Channel"=w563:string, "Reset Value"=w570:string)  [unwired: 6 in, 1 out]
                n212 = case shown="True" w567 {
                  tunnel: w566 -> [_ w592]
                  tunnel: w565 -> [_ w591]
                  tunnel: w561 -> [_ w590]
                  tunnel: w563 -> [w584 w588]
                  tunnel: [w584 w587] -> w562
                  frame False {
                  }
                  frame True {
                    n213 = for {
                      tunnel: w592 -> [w602]
                      tunnel: w591 -> [w600] mode=indexing
                      tunnel: w590 -> [w599]
                      tunnel: [w598] -> w589 mode=indexing
                      tunnel: w588 -> [w595]
                      stop <- w598 continue-if-true
                      n214 = call "SLSC Search Item in Tree Control.vi"("SLSC Output Tree"=w602, "Item Tag"=w600) -> ("Item"=w601:T18)  [unwired: 10 in, 3 out]
                      n215 = call "SLSC Get Items from Tree Control.vi"("Item"=w601) -> ("Datatype"=w593:string, "Type of Channel"=w596:string)  [unwired: 6 in, 3 out]
                      n216 = Equal?(x=w595, y=w596) -> (x = y?=w594:bool)
                      n217 = Equal?(x=w593, y=w599) -> (x = y?=w597:bool)
                      n218 = And(x=w594, y=w597) -> (x .and. y?=w598:bool)
                    }
                    n219 = And Array Elements(Boolean array=w589) -> (logical AND=w585:bool)
                    n220 = Select(t=w588, s=w585, f="Diff" ("t")) -> (s? t:f=w587:string)
                  }
                }
                n221 = Select(t=w570, s=w568, f=w564) -> (s? t:f=w571:string)
                n222 = case shown="Default" w562 {
                  tunnel: w561 -> [w616 _]
                  tunnel: w583 -> [w615 w811]
                  tunnel: w582 -> [w614 w806]
                  tunnel: w581 -> [w613 w812]
                  tunnel: w580 -> [w612 w810]
                  tunnel: w579 -> [w611 w809]
                  tunnel: w578 -> [w610 w808]
                  tunnel: w577 -> [w609 w807]
                  tunnel: w576 -> [w608 w804]
                  tunnel: w575 -> [w607 _]
                  tunnel: w571 -> [w606 _]
                  tunnel: w572 -> [w605 _]
                  tunnel: w569 -> [w604 w803]
                  tunnel: w568 -> [w603 _]
                  frame Default {
                    # "Show the type of control for Writing"
                    n223 = case shown="\"U32\", \"UInt32\"" w616 {
                      selector: w616 -> [w621 w639 w655 w671 w687 w700 w721 w739 w757 w787]
                      tunnel: w615 -> [w625 w647 w663 w679 w694 w713 w731 w748 w756 w786]
                      tunnel: w614 -> [w624 w644 w658 w675 w696 w708 w725 w742 w762 w791]
                      tunnel: w613 -> [w632 w648 w664 w680 w695 w714 w732 w741 w767 w796]
                      tunnel: w612 -> [w631 w640 w662 w678 w693 w712 w730 w747 w766 w795]
                      tunnel: w611 -> [w630 w642 w656 w673 w692 w711 w729 w746 w765 w794]
                      tunnel: w610 -> [w629 w646 w661 w677 w691 w706 w728 w745 w764 w793]
                      tunnel: w609 -> [w628 w641 w660 w672 w690 w710 w727 w744 w763 w792]
                      tunnel: w608 -> [w627 w643 w657 w674 w689 w707 w724 w740 w761 w790]
                      tunnel: w607 -> [_ _ _ _ _ _ _ _ w768 _]
                      tunnel: w606 -> [w620 w638 w654 w670 w686 w699 w720 w738 w759 w788]
                      tunnel: w605 -> [_ _ _ _ _ _ _ _ w758 _]
                      tunnel: w604 -> [w617 w636 w652 w668 w684 w702 w718 w736 w752 w782]
                      tunnel: w603 -> [_ _ _ _ _ _ _ _ _ w778]
                      frame "Bool", "Boolean" {
                        w618 = TRUE ("Visible")
                        n224 = call "SLSC Convert Items - String to Variants.vi"("Datatype"=w621, "Value"=w620) -> ("Value (DBL)"=w619:dbl)  [unwired: 10 in, 3 out]
                        n225 = Build Array(w632, w624, w631, w630, w629, w628, w627) -> (w626:refnum<vi>[])
                        n226 = for {
                          tunnel: w626 -> [w634] mode=indexing
                          n227 = property class="DigNum"(reference=w634, "Visible"=FALSE) -> ()  [unwired: 1 in, 2 out]
                        }
                        n228 = property on="Ring" class="Ring (strict)"("StringsAndValues[]"=T10 [{"String"="False", "Value"=0}, {"String"="True", "Value"=1}] ("Strings And Values []")) -> (error out=w622:errorcluster)  [unwired: 2 in, 1 out]
                        n229 = property class="Ring (strict)"(reference=w625, error in=w622, "Visible"=w618, "Value"=w619) -> ()  [unwired: 2 out]
                        n230 = property class="Bool (strict)"(reference=w617, "Visible"=w618) -> ()  [unwired: 1 in, 2 out]
                      }
                      frame "I8", "Int8" {
                        w635 = TRUE ("Visible")
                        n231 = call "SLSC Convert Items - String to Variants.vi"("Datatype"=w639, "Value"=w638) -> ("Value (DBL)"=w637:dbl)  [unwired: 10 in, 3 out]
                        n232 = Build Array(w648, w647, w641, w643, w646, w642, w644) -> (w645:refnum<vi>[])
                        n233 = for {
                          tunnel: w645 -> [w650] mode=indexing
                          n234 = property class="Num"(reference=w650, "Visible"=FALSE) -> ()  [unwired: 1 in, 2 out]
                        }
                        n235 = property class="DigNum (strict)"(reference=w640, "Visible"=w635, "Value"=w637) -> ()  [unwired: 1 in, 2 out]
                        n236 = property class="Bool (strict)"(reference=w636, "Visible"=w635) -> ()  [unwired: 1 in, 2 out]
                      }
                      frame "I32", "Int32" {
                        w651 = TRUE ("Visible")
                        n237 = call "SLSC Convert Items - String to Variants.vi"("Datatype"=w655, "Value"=w654) -> ("Value (DBL)"=w653:dbl)  [unwired: 10 in, 3 out]
                        n238 = Build Array(w664, w663, w662, w657, w661, w660, w658) -> (w659:refnum<vi>[])
                        n239 = for {
                          tunnel: w659 -> [w666] mode=indexing
                          n240 = property class="Num"(reference=w666, "Visible"=FALSE) -> ()  [unwired: 1 in, 2 out]
                        }
                        n241 = property class="DigNum (strict)"(reference=w656, "Visible"=w651, "Value"=w653) -> ()  [unwired: 1 in, 2 out]
                        n242 = property class="Bool (strict)"(reference=w652, "Visible"=w651) -> ()  [unwired: 1 in, 2 out]
                      }
                      frame "U8", "UInt8" {
                        w667 = TRUE ("Visible")
                        n243 = call "SLSC Convert Items - String to Variants.vi"("Datatype"=w671, "Value"=w670) -> ("Value (DBL)"=w669:dbl)  [unwired: 10 in, 3 out]
                        n244 = Build Array(w680, w679, w678, w674, w677, w673, w675) -> (w676:refnum<vi>[])
                        n245 = for {
                          tunnel: w676 -> [w682] mode=indexing
                          n246 = property class="Num"(reference=w682, "Visible"=FALSE) -> ()  [unwired: 1 in, 2 out]
                        }
                        n247 = property class="DigNum (strict)"(reference=w672, "Visible"=w667, "Value"=w669) -> ()  [unwired: 1 in, 2 out]
                        n248 = property class="Bool (strict)"(reference=w668, "Visible"=w667) -> ()  [unwired: 1 in, 2 out]
                      }
                      frame "U32", "UInt32" {
                        w683 = TRUE ("Visible")
                        n249 = Build Array(w695, w694, w693, w692, w691, w690, w689) -> (w688:refnum<vi>[])
                        n250 = call "SLSC Convert Items - String to Variants.vi"("Datatype"=w687, "Value"=w686) -> ("Value (DBL)"=w685:dbl)  [unwired: 10 in, 3 out]
                        n251 = for {
                          tunnel: w688 -> [w698] mode=indexing
                          n252 = property class="Num"(reference=w698, "Visible"=FALSE) -> ()  [unwired: 1 in, 2 out]
                        }
                        n253 = property class="DigNum (strict)"(reference=w696, "Visible"=w683, "Value"=w685) -> ()  [unwired: 1 in, 2 out]
                        n254 = property class="Bool (strict)"(reference=w684, "Visible"=w683) -> ()  [unwired: 1 in, 2 out]
                      }
                      frame "I64", "Int64" {
                        w701 = TRUE ("Visible")
                        n255 = call "SLSC Convert Items - String to Variants.vi"("Datatype"=w700, "Value"=w699) -> ("Value"=w705:variant)  [unwired: 10 in, 3 out]
                        n256 = Build Array(w714, w713, w712, w711, w707, w710, w708) -> (w709:refnum<vi>[])
                        n257 = for {
                          tunnel: w709 -> [w716] mode=indexing
                          n258 = property class="Num"(reference=w716, "Visible"=FALSE) -> ()  [unwired: 1 in, 2 out]
                        }
                        n259 = Variant To Data(type=i64 0, Variant=w705) -> (data=w703:i64)  [unwired: 1 in, 1 out]
                        n260 = property class="DigNum (strict)"(reference=w706, "Visible"=w701, "Value"=w703) -> ()  [unwired: 1 in, 2 out]
                        n261 = property class="Bool (strict)"(reference=w702, "Visible"=w701) -> ()  [unwired: 1 in, 2 out]
                      }
                      frame "U64", "UInt64" {
                        w717 = TRUE ("Visible")
                        n262 = call "SLSC Convert Items - String to Variants.vi"("Datatype"=w721, "Value"=w720) -> ("Value"=w719:variant)  [unwired: 10 in, 3 out]
                        n263 = Build Array(w732, w731, w730, w729, w728, w727, w725) -> (w726:refnum<vi>[])
                        n264 = for {
                          tunnel: w726 -> [w734] mode=indexing
                          n265 = property class="Num"(reference=w734, "Visible"=FALSE) -> ()  [unwired: 1 in, 2 out]
                        }
                        n266 = Variant To Data(type=u64 0, Variant=w719) -> (data=w722:u64)  [unwired: 1 in, 1 out]
                        n267 = property class="Bool (strict)"(reference=w718, "Visible"=w717) -> ()  [unwired: 1 in, 2 out]
                        n268 = property class="DigNum (strict)"(reference=w724, "Visible"=w717, "Value"=w722) -> ()  [unwired: 1 in, 2 out]
                      }
                      frame "DBL", "Double" {
                        w735 = TRUE ("Visible")
                        n269 = call "SLSC Convert Items - String to Variants.vi"("Datatype"=w739, "Value"=w738) -> ("Value (DBL)"=w737:dbl)  [unwired: 10 in, 3 out]
                        n270 = Build Array(w740, w748, w747, w746, w745, w744, w742) -> (w743:refnum<vi>[])
                        n271 = for {
                          tunnel: w743 -> [w750] mode=indexing
                          n272 = property class="Num"(reference=w750, "Visible"=FALSE) -> ()  [unwired: 1 in, 2 out]
                        }
                        n273 = property class="DigNum (strict)"(reference=w741, "Visible"=w735, "Value"=w737) -> ()  [unwired: 1 in, 2 out]
                        n274 = property class="Bool (strict)"(reference=w736, "Visible"=w735) -> ()  [unwired: 1 in, 2 out]
                      }
                      frame Default {
                        n275 = Build Array(w767, w766, w765, w764, w763, w762, w761) -> (w760:refnum<vi>[])
                        n276 = call "SLSC Search and Convert ENUM Value by Name.vi"("Enum Strings"=w758, "enums"=w768, "Value"=w759, "Datatype Name"=w757) -> ("Enum"=w754:T3, "Datatype found?"=w751:bool, "Value"=w755:i32)  [unwired: 5 in]
                        n277 = for {
                          tunnel: w760 -> [w770] mode=indexing
                          n278 = property class="DigNum"(reference=w770, "Visible"=FALSE) -> ()  [unwired: 1 in, 2 out]
                        }
                        n279 = case shown="False" w751 {
                          tunnel: w754 -> [_ w773]
                          frame False {
                            # "Datatype not found: hide all controls"
                          }
                          frame True {
                            # "Show Ring control for custom datatype"
                            n280 = Unbundle By Name(w773) -> ("values"=w772:T19)
                            n281 = for {
                              tunnel: w772 -> [w777] mode=indexing
                              tunnel: [w774] -> w771 mode=indexing
                              n282 = Unbundle(w777) -> ("name"=w776:string, "value"=w775:i32)  [unwired: 1 out]
                              n283 = Bundle("name"=w776, "value"=w775) -> (w774:cluster{"name":string, "value":i32})  [unwired: 1 in]
                            }
                            n284 = property on="Ring" class="Ring (strict)"("StringsAndValues[]"=w771) -> ()  [unwired: 2 in, 2 out]
                          }
                        }
                        n285 = property class="Ring (strict)"(reference=w756, "Visible"=w751, "Value"=w755) -> (error out=w753:errorcluster)  [unwired: 1 in, 1 out]
                        n286 = property class="Bool (strict)"(reference=w752, error in=w753, "Visible"=w751) -> ()  [unwired: 2 out]
                      }
                      frame "Command" {
                        w781 = TRUE
                        n287 = Build Array(w796, w795, w794, w793, w792, w791, w790) -> (w789:refnum<vi>[])
                        n288 = call "SLSC Command Enum Constant.vi"("Option on Reset?"=w778) -> ("Array"=w783:T3[])  [unwired: 10 in, 4 out]
                        n289 = for {
                          tunnel: w789 -> [w802] mode=indexing
                          n290 = property class="DigNum"(reference=w802, "Visible"=FALSE) -> ()  [unwired: 1 in, 2 out]
                        }
                        n291 = call "SLSC Search and Convert ENUM Value by Name.vi"("enums"=w783, "Value"=w788, "Datatype Name"=w787) -> ("Enum"=w784:T3, "Value"=w785:i32)  [unwired: 6 in, 1 out]
                        n292 = Unbundle By Name(w784) -> ("values"=w780:T19)
                        n293 = for {
                          tunnel: w780 -> [w800] mode=indexing
                          tunnel: [w797] -> w779 mode=indexing
                          n294 = Unbundle(w800) -> ("name"=w799:string, "value"=w798:i32)  [unwired: 1 out]
                          n295 = Bundle("name"=w799, "value"=w798) -> (w797:cluster{"name":string, "value":i32})  [unwired: 1 in]
                        }
                        n296 = property on="Ring" class="Ring (strict)"("StringsAndValues[]"=w779) -> ()  [unwired: 2 in, 2 out]
                        n297 = property class="Ring (strict)"(reference=w786, "Visible"=w781, "Value"=w785) -> ()  [unwired: 1 in, 2 out]
                        n298 = property class="Bool (strict)"(reference=w782, "Visible"=w781) -> ()  [unwired: 1 in, 2 out]
                      }
                    }
                  }
                  frame "Diff", "Don't Read", "Multi " {
                    # "Remove the Control Change"
                    n299 = Build Array(w812, w811, w810, w809, w808, w807, w806, w804, w803) -> (w805:refnum<vi>[])
                    n300 = for {
                      tunnel: w805 -> [w814] mode=indexing
                      n301 = property class="Ctl"(reference=w814, "Visible"=FALSE) -> ()  [unwired: 1 in, 2 out]
                    }
                  }
                }
              }
              frame True {
                n302 = Build Array(w824, w823, w822, w821, w820, w819, w818, w817, w815) -> (w816:refnum<vi>[])
                n303 = for {
                  tunnel: w816 -> [w826] mode=indexing
                  n304 = property class="Ctl"(reference=w826, "Visible"=FALSE) -> ()  [unwired: 1 in, 2 out]
                }
              }
            }
          }
          event "Modify Reset Value?": Value Change {
            n305 = event-data() -> ("NewVal"=w830:bool)  [unwired: 6 out]
            n306 = control-ref of="Property tree"() -> (w831:refnum<vi>)
            n307 = Select(t=2 ("Active Cell:Active Column Number"), s=w830, f=1 ("Active Cell:Active Column Number")) -> (s? t:f=w829:i32)
            n308 = call "SLSC Change Color of Table Header.vi"("error in (no error)"=w828, "Active Cell:Active Column Number"=w829, "TreeControl in"=w831) -> ("error out"=w827:errorcluster)  [unwired: 8 in]
            n309 = local read "Property tree"() -> (w834:string[])
            n310 = property on="Property tree" class="Tree (strict)"("Val(Sgnl)"=w834) -> ()  [unwired: 2 in, 2 out]
          }
          event "Property tree": Mouse Down {
            w841 = 2 ("upper limit")
            # "-3 means no highlilght"
            # "Highlight the Default Value\nand the Reset Value only"
            n311 = event-data() -> ("Coords"=w852:T20)  [unwired: 1 out]
            n312 = invoke on="Property tree" class="Tree (strict)" method="Point To Row Column"("Point"=w852) -> ("Col"=w840:i32)  [unwired: 7 in, 7 out]
            n313 = In Range and Coerce(upper limit=w841, x=w840, lower limit=1) -> (coerced(x)=w844:i32, In Range?=w845:bool)
            n314 = Equal?(x=w840, y=w841) -> (x = y?=w839:bool)
            n315 = local write "Modify Reset Value?"(w839) -> ()
            n316 = Select(t=w844, s=w845, f=-3) -> (s? t:f=w842:i32)
            n317 = control-ref of="Property tree"() -> (w849:refnum<vi>)
            n318 = call "SLSC Change Color of Table Header.vi"("error in (no error)"=w848, "Active Cell:Active Column Number"=w842, "TreeControl in"=w849) -> ("error out"=w847:errorcluster)  [unwired: 8 in]
          }
          event "Loop rate": Value Change {
            n319 = event-data() -> ()  [unwired: 2 out]
            n320 = call "SLSC Set Sampling Time.vi"("error in (no error)"=w856, "Loop rate"="Loop rate", "Section Ref in"=w857) -> ("error out"=w861:errorcluster)  [unwired: 7 in, 1 out]
          }
          event "Refresh page": Value Change {
            # "The main reason of this page is to allow a \"chassis\" to placed online\nafter this page is on. Also, it has a longer timeout, so if the 0.5 is \nnot sufficient (or the chassis does not respond), then you can click\nrefresh and this should be able to reach the chassis (I use 4 for now)"
            # "Refresh is also used to refresh the main page data,\njust in case the asynch nature of VS don't work.\nThis code can be removed in the future if this is not \nnecessary anymore..."
            n321 = event-data() -> ()  [unwired: 7 out]
            n322 = flat-sequence {
              tunnel: [w903] -> w869
              tunnel: w897 -> [w904]
              frame #0 {
                # "Force the button down..."
                n323 = call "SLSC Disable Buttons.vi"("error in (no error)"=w904) -> ("error out"=w903:errorcluster)  [unwired: 10 in]
                n324 = local write "Refresh page"(TRUE ("Connection")) -> ()
              }
            }
            n325 = global read "Constants.vi" "Capabilities"() -> (w891:string)
            n326 = call "SLSC Get Capabilities from Custom Device.vi"("Property Name"=w891, "error in (no error)"=w869, "Device Item Ref in"=w890) -> ("error out"=w870:errorcluster, "data"=w882:T2, "Item Ref out"=w883:T1)  [unwired: 3 in, 3 out]
            n327 = global read "Constants.vi" "SLSCChannelPath"() -> (w889:string)
            n328 = call "SLSC Get All Channels.vi"("SLSCChannelPath"=w889, "error in (no error)"=w870, "Item Ref in"=w883) -> ("error out"=w886:errorcluster, "Channel Values"=w888:dbl[], "TreeItem Channels"=w887:string[], "Item Ref out"=w874:T1)  [unwired: 5 in]
            n329 = control-ref of="Property tree"() -> (w885:refnum<vi>)
            n330 = call "SLSC Create Tree Control from EDS datatype.vi"("Property Tree"=w885, "error in (no error)"=w886, "Channel Values"=w888, "Properties to enable"=w887, "SLSC EDS module"=w882) -> ("error out"=w868:errorcluster, "Enum Strings"=w871:cluster{"name":string, string}[], "Enums"=w872:T3[], "SLSC Output Tree"=w873:T9)  [unwired: 3 in]
            n331 = call "SLSC Get SLSC name from Custom Device Ref.vi"("connect timeout"=4.0, "error in (no error)"=w869, "Wait for mDSN?"=TRUE, "Item Ref in"=w890) -> ("error out"=w894:errorcluster, "SLSC Module Name"=w898:string)  [unwired: 4 in, 2 out]
            n332 = call "SLSC Update Default Values in Tree.vi"("error in (no error)"=w868, "SLSC Output Tree"=w873, "SLSC EDS module in"=w882) -> ("error out"=w867:errorcluster, "SLSC EDS module out"=w884:T2)  [unwired: 7 in]
            n333 = global read "Constants.vi" "Device.Error.message"() -> (w895:string)
            n334 = call "SLSC Get Channel Properties.vi"("Node Ptr"=w874, "error in (no error)"=w867) -> ("Loop time (ms)"=w881:u32, "Description"=w879:string, "Module Number"=w876:i32, "Name"=w880:string, "Device Version"=w875:string, "Default Value"=w877:bool, "Reset Value"=w878:bool, "error out"=w865:errorcluster)  [unwired: 5 in, 1 out]
            n335 = local write "Loop rate"(w881) -> ()
            n336 = local write "Description"(w879) -> ()
            n337 = local write "Slot Number"(w876) -> ()
            n338 = local write "Name"(w880) -> ()
            n339 = local write "CD Version"(w875) -> ()
            n340 = local write "Apply Reset"(w878) -> ()
            n341 = local write "Apply Default"(w877) -> ()
            n342 = Merge Errors(w894, w865) -> (w866:errorcluster)
            n343 = Select(t=w895, s=w894, f=w898) -> (s? t:f=w899:string)
            n344 = call "SLSC Enable Buttons for Online Action.vi"("error in (no error)"=w894) -> ()  [unwired: 11 in]
            n345 = local write "SLSC Device Name"(w899) -> ()
            n346 = call <vilib>:"Simple Error Handler.vi"("error in (no error)"=w866) -> ("error out"=w900:errorcluster)  [unwired: 1 in, 7 out]
            n347 = call <vilib>:"Clear Errors.vi"("error in (no error)"=w900) -> ("error out"=w892:errorcluster)  [unwired: 1 in, 5 out]
            n348 = call "SLSC Enable Buttons.vi"("error in (no error)"=w892, "data"=w884) -> ()  [unwired: 10 in]
            n349 = flat-sequence {
              tunnel: [w901] -> w896
              tunnel: w892 -> [w901]
              frame #0 {
                # "... until the whole page is done"
                n350 = local write "Refresh page"(FALSE ("Connection")) -> ()
              }
            }
          }
          event "State": Value Change {
            n351 = event-data() -> ("NewVal"=w906:u16)  [unwired: 6 out]
            n352 = property on="State" class="Ring (strict)"() -> ("Strings []"=w907:string[])  [unwired: 2 in, 2 out]
            n353 = Index Array(array=w907, index=w906) -> (element=→"Custom Device State":string)
          }
          event "Help Button": Value Change {
            n354 = event-data() -> ("NewVal"=w918:bool)  [unwired: 1 out]
            n355 = property on="SHDocVw.IWebBrowser" class="AXCont"("Visible"=w918) -> ()  [unwired: 2 in, 2 out]
          }
          event "Apply Reset", "Apply Default": Value Change {
            n356 = event-data() -> ()  [unwired: 7 out]
            n357 = call "SLSC Set Default-Reset Value.vi"("error in (no error)"=w926, "Apply Reset"="Apply Reset", "Apply Default"="Apply Default", "Section Ref in"=w927) -> ("error out"=w920:errorcluster)  [unwired: 6 in, 1 out]
          }
          event "Name": Value Change {
            n358 = event-data() -> ()  [unwired: 2 out]
            n359 = call <vilib>:"NI VeriStand - Rename Custom Device Item.vi"("error in (no error)"=w936, "New Name"="Name", "Item Ref in"=w934) -> ("error out"=w935:errorcluster)  [unwired: 1 in, 7 out]
          }
          event "Description": Value Change {
            n360 = event-data() -> ()  [unwired: 2 out]
            n361 = call <vilib>:"NI VeriStand - Set Item Description.vi"("error in (no error)"=w943, "Description"="Description", "Item Ref in"=w944) -> ("error out"=w942:errorcluster)  [unwired: 8 out]
          }
          event "Remove", "Add": Value Change {
            # "Remove non-critical error. Keep pop-up\nin case you need to debug."
            # "Need to update\nicons in the controls"
            n362 = event-data() -> ()  [unwired: 2 out]
            n363 = global read "Constants.vi" "Command Channel"() -> (w960:string)
            n364 = local read "Property tree"() -> (w947:string[])
            n365 = global read "Constants.vi" "Physical Channels"() -> (w959:string)
            n366 = global read "Constants.vi" "Properties"() -> (w961:string)
            n367 = call "SLSC Add or Remove Channels.vi"("Section Ref in"=w955, "Properties"=w961, "Command Channel"=w960, "Physical Channels"=w959, "Property tree"=w947, "Add or Remove"="Add", "SLSC EDS module in"=w958, "error in (no error)"=w945, "Enums"=w956) -> ("Section Ref out"=w953:T1, "error out"=w954:errorcluster)  [unwired: 5 in]
            n368 = control-ref of="Property tree"() -> (w949:refnum<vi>)
            n369 = global read "Constants.vi" "SLSCChannelPath"() -> (w948:string)
            n370 = call "SLSC Refresh Tree Control.vi"("SLSCChannelPath"=w948, "Update Only?"=TRUE, "enums"=w956, "TreeControl in"=w949, "error in (no error)"=w954, "SLSC Output Tree"=w963, "Item Ref in"=w953) -> ("error out"=w951:errorcluster)  [unwired: 3 in, 1 out]
            n371 = disable-structure shown="Enabled" {
              disable-tunnel: w951 -> [w965 w966]
              disable-tunnel: [w964 w966] -> w950
              frame Disabled {
                n372 = call <vilib>:"Simple Error Handler.vi"("error in (no error)"=w965) -> ("error out"=w964:errorcluster)  [unwired: 4 in, 4 out]
              }
              frame Enabled {
              }
            }
            n373 = flat-sequence {
              tunnel: w954 -> [w967]
              tunnel: [w967] -> w946
              frame #0 {
                w968 = FALSE ("Remove")
                n374 = local write "Remove"(w968) -> ()
                n375 = local write "Add"(w968) -> ()
              }
            }
            n376 = call <vilib>:"Clear Errors.vi"("error in (no error)"=w950) -> ()  [unwired: 1 in, 6 out]
          }
          event "Ring", "I64", "U64", "U32", "I32", "U8", "I8", "DBL": Value Change {
            n377 = event-data() -> ("NewVal"=w981:variant)  [unwired: 1 out]
            n378 = global read "Constants.vi" "Command Channel"() -> (w979:string)
            n379 = local read "Property tree"() -> (w983:string[])
            n380 = control-ref of="Property tree"() -> (w982:refnum<vi>)
            n381 = global read "Constants.vi" "Properties"() -> (w980:string)
            n382 = local read "Modify Reset Value?"() -> (w985:bool)
            n383 = call "SLSC Update Values in Tree Control.vi"("Section Ref in"=w969, "TreeControl in"=w982, "Properties"=w980, "Command Channel"=w979, "Property tree in"=w983, "NewVal"=w981, "SLSC Output Tree"=w984, "error in (no error)"=w986, "Enums"=w975, "Enum Strings"=w976, "Modify Reset Value?"=w985) -> ("SLSC Output Tree Out"=w971:T9, "error out"=w977:errorcluster)  [unwired: 3 in]
            n384 = global read "Constants.vi" "Capabilities"() -> (w974:string)
            n385 = call "SLSC Update Default Values in Tree.vi"("error in (no error)"=w977, "SLSC Output Tree"=w971, "SLSC EDS module in"=w978) -> ("error out"=w973:errorcluster, "SLSC EDS module out"=w970:T2)  [unwired: 7 in]
            n386 = call-poly <vilib>:"NI VeriStand - Set Item Property.vi"("error in (no error)"=w973, "Value"=w970, "Property Name"=w974, "Item Ref in"=w969) -> ("error out"=w972:errorcluster)  [unwired: 5 in, 2 out]
          }
        }
        n387 = call <vilib>:"Simple Error Handler.vi"("error in (no error)"=w93) -> ("error out"=w103:errorcluster)  [unwired: 1 in, 7 out]
        n388 = call <vilib>:"Clear Errors.vi"("error in (no error)"=w103) -> ("error out"=w102:errorcluster)  [unwired: 1 in, 5 out]
      }
      n389 = Unregister For Events(event registration refnum=w91, error in=w90) -> (error out=w89:errorcluster)
    }
    frame Error {
      # "#Todo: Removing errors that\ncould happen if you change\nfrom one page to another. This \nerror can make the VS 2017 driver to break. \nBut this is just a workaround... maybe we \nshould invest more time to understand why\nthis happen and how to fix it."
      n390 = call <vilib>:"Clear Errors.vi"("error in (no error)"=w989, "specific error code to clear (0: all)"=1055) -> ("error out"=w988:errorcluster)  [unwired: 4 in, 1 out]
      n391 = call <vilib>:"Simple Error Handler.vi"("error in (no error)"=w988) -> ("error out"=w991:errorcluster)  [unwired: 1 in, 7 out]
      n392 = call <vilib>:"Clear Errors.vi"("error in (no error)"=w991) -> ("error out"=w990:errorcluster)  [unwired: 1 in, 5 out]
    }
  }
  n393 = invoke class="VI" method="FP.Close"(error in=w52) -> (error out=w51:errorcluster)  [unwired: 2 in, 2 out]
  n394 = call <vilib>:"NI VeriStand - Signal When Ready for Shutdown.vi"("error in (no error)"=w51) -> ("error out"=→"error out":errorcluster)  [unwired: 10 out]
